vi "Status Manager Init.vi"(8 "error in (no error)":errorcluster, 11 "N (1)":i32=1) -> (0 "error out":errorcluster, 3 "Status References":T1[](array[typedef]))   [LabVIEW 2019, in "Status.lvlib"]
uses:
  Status.lvlib
  Ctl/control.ctl
  Ctl/State.ctl
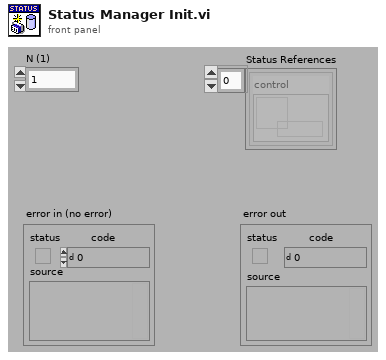
[diagram p1: front panel]
types:
  T1 = typedef "Status.lvlib/control.ctl" = cluster{"control":refnum<data-value>}
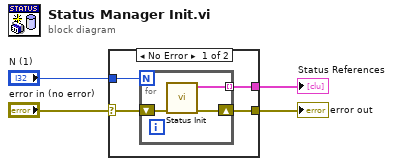
[diagram p0: block diagram]
diagram:
  n1 = case shown="No Error" "error in (no error)" {
    selector: "error in (no error)" -> [w7 w12]
    tunnel: [w8 _] -> w4
    tunnel: "N (1)" -> [w6 _]
    tunnel: [w5 w12] -> w1
    frame No Error {
      n2 = for {
        N: w6 -> [_]
        shift-right: [w10] -> w5
        shift-left: w7 -> [w11]
        tunnel: [w9] -> w8 mode=indexing
        n3 = call "Status Init.vi"("error in (no error)"=w11) -> ("error out"=w10:errorcluster, "Status Reference"=w9:T1)  [unwired: 9 in]
      }
    }
    frame Error {
    }
  }
  "error out" <- w1
  "Status References" <- w4
